vi "Set Stopped.vi"(8 "error in (no error)":errorcluster {"code" format="Error %.0f"}, 10 "Process":string, 11 "Progress Bar UI In":refnum<class "Progress Bar UI.lvclass">) -> (0 "error out":errorcluster {"code" format="Error %.0f"}, 3 "Progress Bar UI Out":refnum<class "Progress Bar UI.lvclass">)   [LabVIEW 2023, in "Progress Bar UI.lvclass"]
uses:
  Progress Bar UI.lvclass
  Progress Bar UI.lvclass/Progress Bar UI.ctl
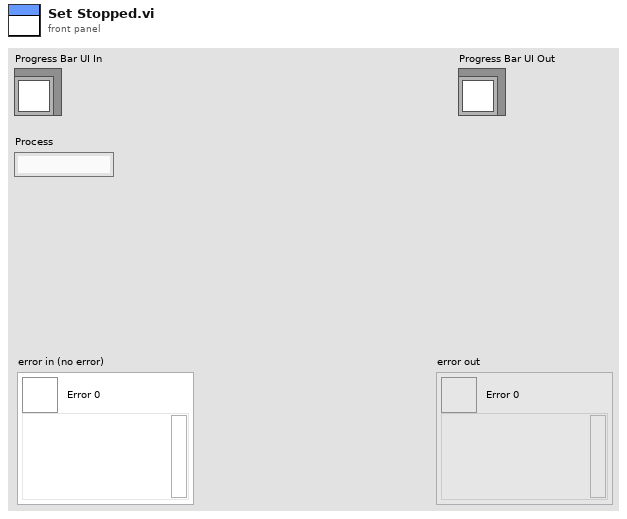
[diagram p1: front panel]
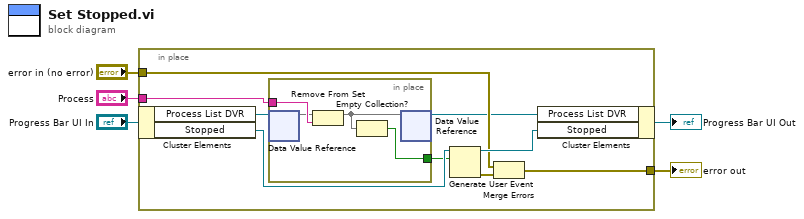
[diagram p0: block diagram]
diagram:
  n1 = in-place {
    in-place-border: "error in (no error)" -> [w10]
    in-place-border: [w11] -> w3
    in-place-border: "Process" -> [w9]
    n2 = in-place-cluster #1("Progress Bar UI In") -> ("Process List DVR"=w8:refnum<data-value>, "Stopped"=w14:refnum<user-event>)
    n3 = in-place {
      in-place-border: w9 -> [w18]
      in-place-border: [w16] -> w7
      n4 = in-place-dvr #2(w8) -> (w17:set{string})  [unwired: 1 out]
      n5 = Remove From Set(10:w18, 11:w17) -> (3:w15:set{string})  [unwired: 1 out]
      n6 = Empty Collection?(1:w15) -> (0:w16:bool)
      n7 = in-place-dvr #2(w15) -> (w6:refnum<data-value>)  [unwired: 1 out]
    }
    n8 = Generate User Event(user event=w14, event data cluster=w7) -> (user event out=w13:refnum<user-event>, error out=w12:errorcluster)  [unwired: 2 in]
    n9 = Merge Errors(w10, w12) -> (w11:errorcluster)
    n10 = in-place-cluster #1("Process List DVR"=w6, "Stopped"=w13) -> (→"Progress Bar UI Out":refnum<class "Progress Bar UI.lvclass">)
  }
  "error out" <- w3
